vi "Find and Validate Measurement and Device Selection.vi"(8 "error in (no error)":errorcluster, 9 "Device Names":string[](array[string]), 10 "Measurement Name":string, 11 "Controller in":refnum<class "Controller.lvclass">) -> (0 "error out":errorcluster, 1 "Hardware Objects":refnum<class "Hardware.lvclass">[](array[class]), 2 "Measurement out":refnum<class "Measurement.lvclass">, 3 "Controller out":refnum<class "Controller.lvclass">)   [LabVIEW 2015, in "Controller Actor.lvlib" / "Controller.lvclass"]
uses:
  Controller.lvclass
  Hardware/Hardware.lvclass
  Measurement Actor/Measurement.lvclass
panel:
  # "INPUTS"
  # "OUTPUTS"
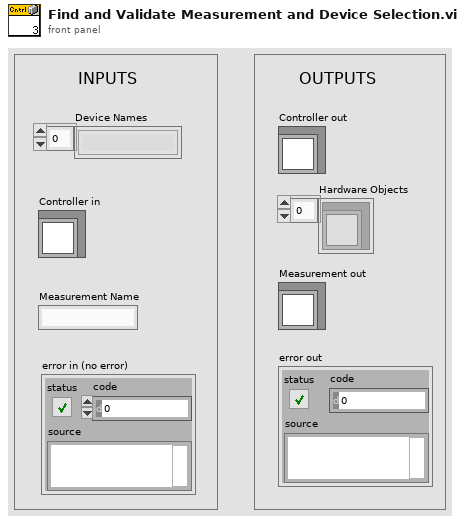
[diagram p1: front panel]
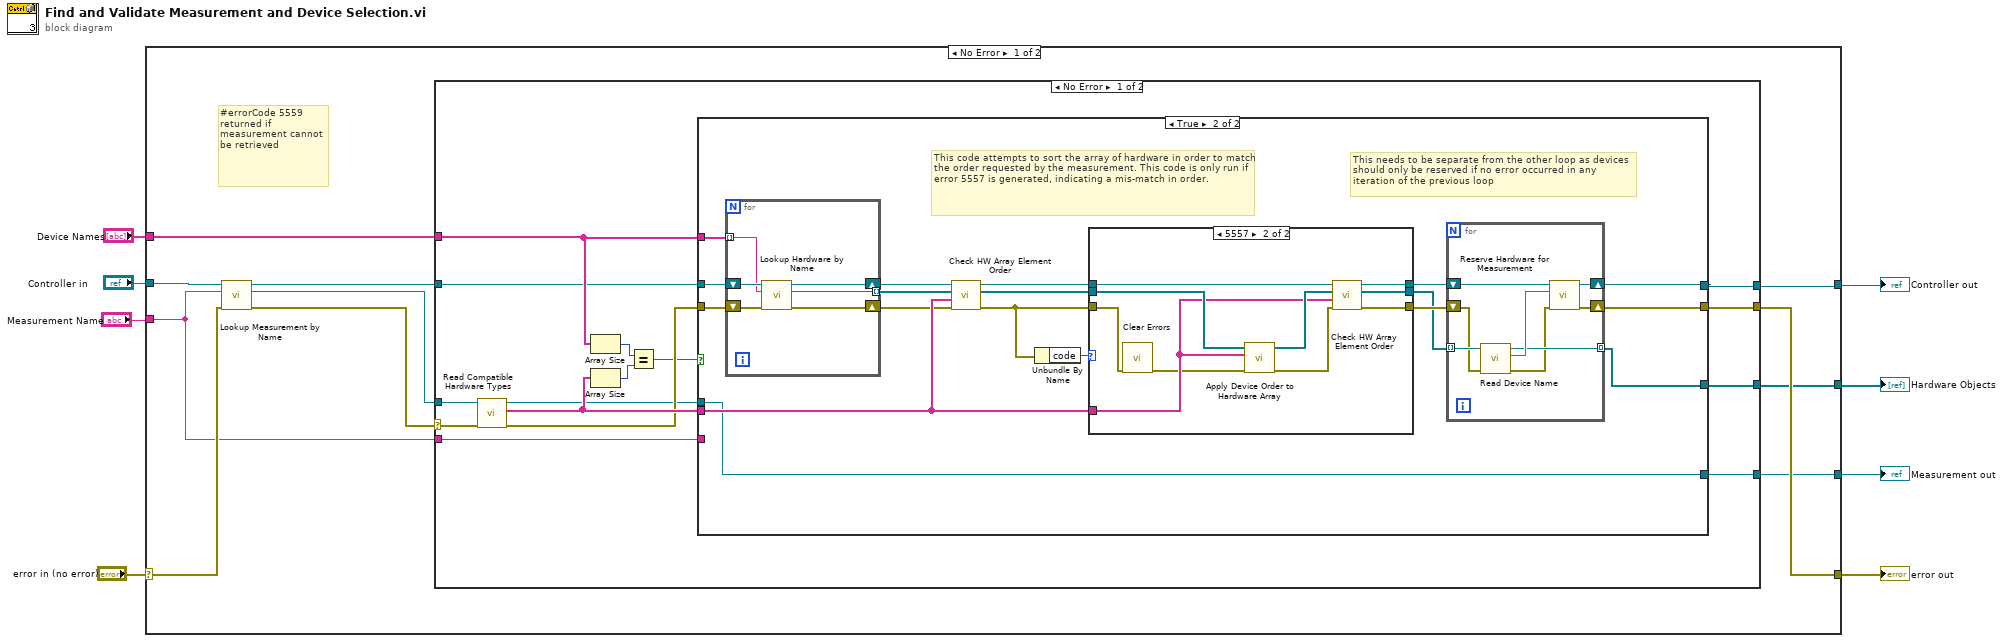
[diagram p0: block diagram]
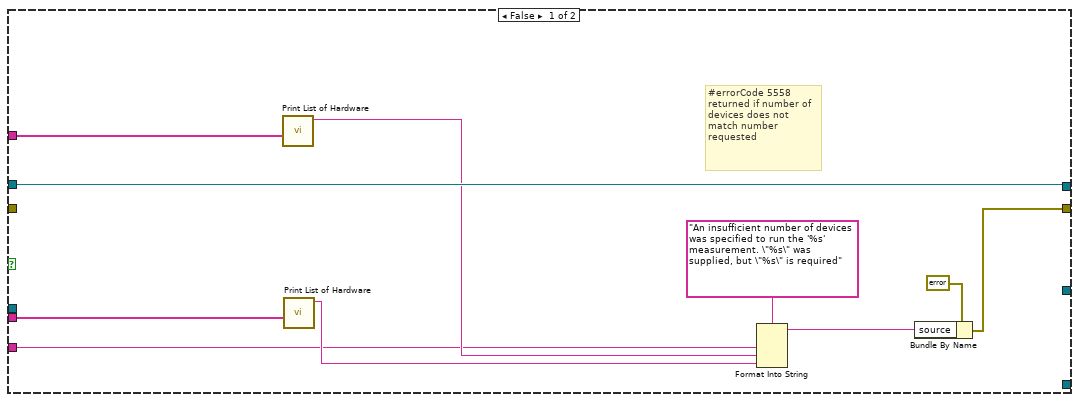
[diagram p2: hidden frame]
diagram:
  n1 = case shown="No Error" "error in (no error)" {
    selector: "error in (no error)" -> [w13 w92]
    tunnel: [w19 w92] -> w8
    tunnel: [w18 w93] -> w7
    tunnel: [w17 _] -> w6
    tunnel: "Controller in" -> [w15 w93]
    tunnel: "Device Names" -> [w16 _]
    tunnel: "Measurement Name" -> [w10 _]
    tunnel: [w11 _] -> w2
    frame No Error {
      # "#errorCode 5559 returned if measurement cannot be retrieved"
      n2 = call "Lookup Measurement by Name.vi"("error in (no error)"=w13, "Measurement Name"=w10, "Controller in"=w15) -> ("error out"=w9:errorcluster, "Measurement.lvclass"=w12:refnum<class "Measurement.lvclass">, "Controller out"=w14:refnum<class "Controller.lvclass">)  [unwired: 5 in, 1 out]
      n3 = case shown="No Error" w9 {
        selector: w9 -> [w20 w91]
        tunnel: [w34 w91] -> w19
        tunnel: [w33 w90] -> w18
        tunnel: [w32 _] -> w17
        tunnel: w16 -> [w31 _]
        tunnel: w14 -> [w25 w90]
        tunnel: w12 -> [w24 _]
        tunnel: [w22 _] -> w11
        tunnel: w10 -> [w21 _]
        frame No Error {
          n4 = call-dynamic "Read Compatible Hardware Types.vi"("error in (no error)"=w20, "Measurement in"=w24) -> ("error out"=w29:errorcluster, "Compatible Hardware Types"=w30:string[], "Measurement out"=w23:refnum<class "Measurement.lvclass">)  [unwired: 7 in]
          n5 = Array Size(array=w31) -> (size(s)=w27:i32)
          n6 = Array Size(array=w30) -> (size(s)=w26:i32)
          n7 = Equal?(x=w27, y=w26) -> (x = y?=w28:bool)
          n8 = case shown="True" w28 {
            tunnel: [w36 w62] -> w34
            tunnel: [w44 w61] -> w33
            tunnel: [_ w49] -> w32
            tunnel: w29 -> [_ w54]
            tunnel: w25 -> [w44 w56]
            tunnel: w31 -> [w43 w57]
            tunnel: w30 -> [w42 w59]
            tunnel: w23 -> [_ w58]
            tunnel: [_ w58] -> w22
            tunnel: w21 -> [w35 _]
            frame False {
              # "#errorCode 5558 returned if number of devices does not match number requested"
              n9 = call "Print List of Hardware.vi"("Device Names"=w43) -> ("String"=w40:string)  [unwired: 10 in]
              n10 = call "Print List of Hardware.vi"("Device Names"=w42) -> ("String"=w39:string)  [unwired: 10 in]
              n11 = Format Into String(format string="An insufficient number of devices was specified to run the '%s' measurement. \"%s\" was supplied, but \"%s\" is required", w35, w40, w39) -> (resulting string=w37:string)  [unwired: 2 in, 1 out]
              n12 = Bundle By Name(cluster=errorcluster {"status"=TRUE, "code"=5558, "source"=""} ("error out"), "source"=w37) -> (w36:errorcluster)
            }
            frame True {
              # "This code attempts to sort the array of hardware in order to match the order requested by the measurement. This code is only run if error 5557 is generated, indicating a mis-match in order."
              # "This needs to be separate from the other loop as devices\nshould only be reserved if no error occurred in any\niteration of the previous loop"
              n13 = for {
                tunnel: w57 -> [w80] mode=indexing
                shift-right: [w79] -> w55
                shift-left: w56 -> [w81]
                shift-right: [w77] -> w53
                shift-left: w54 -> [w78]
                tunnel: [w76] -> w52 mode=indexing
                n14 = call "Lookup Hardware by Name.vi"("error in (no error)"=w78, "Device Name"=w80, "Controller in"=w81) -> ("error out"=w77:errorcluster, "Hardware.lvclass"=w76:refnum<class "Hardware.lvclass">, "Controller out"=w79:refnum<class "Controller.lvclass">)  [unwired: 6 in]
              }
              n15 = call "Check HW Array Element Order.vi"("error in (no error)"=w53, "Compatible Hardware Types"=w59, "Array of Hardware in"=w52, "Controller in"=w55) -> ("error out"=w47:errorcluster, "Array of Hardware out"=w48:refnum<class "Hardware.lvclass">[], "Controller out"=w45:refnum<class "Controller.lvclass">)  [unwired: 5 in]
              n16 = Unbundle By Name(w47) -> ("code"=w46:i32)
              n17 = case shown="5557" w46 {
                tunnel: w59 -> [_ w71]
                tunnel: w48 -> [w64 w75]
                tunnel: [w65 w68] -> w51
                tunnel: w47 -> [w65 w66]
                tunnel: w45 -> [w63 w74]
                tunnel: [w63 w73] -> w60
                tunnel: [w64 w70] -> w50
                frame Default {
                }
                frame 5557 {
                  n18 = call <vilib>:"Clear Errors.vi"("error in (no error)"=w66) -> ("error out"=w67:errorcluster)  [unwired: 5 in, 1 out]
                  n19 = call "Apply Device Order to Hardware Array.vi"("error in (no error)"=w67, "Compatible Hardware Types"=w71, "Array of Hardware in"=w75) -> ("error out"=w69:errorcluster, "Array"=w72:refnum<class "Hardware.lvclass">[])  [unwired: 7 in]
                  n20 = call "Check HW Array Element Order.vi"("error in (no error)"=w69, "Compatible Hardware Types"=w71, "Array of Hardware in"=w72, "Controller in"=w74) -> ("error out"=w68:errorcluster, "Array of Hardware out"=w70:refnum<class "Hardware.lvclass">[], "Controller out"=w73:refnum<class "Controller.lvclass">)  [unwired: 5 in]
                }
              }
              n21 = for {
                shift-right: [w88] -> w61
                shift-left: w60 -> [w89]
                shift-right: [w87] -> w62
                shift-left: w51 -> [w83]
                tunnel: w50 -> [w86] mode=indexing
                tunnel: [w84] -> w49 mode=indexing
                n22 = call "Read Device Name.vi"("error in (no error)"=w83, "Analog in"=w86) -> ("error out"=w82:errorcluster, "Device Name"=w85:string, "Analog out"=w84:refnum<class "Hardware.lvclass">)  [unwired: 7 in]
                n23 = call "Reserve Hardware for Measurement.vi"("error in (no error)"=w82, "Hardware to Reserve"=w85, "Controller in"=w89) -> ("error out"=w87:errorcluster, "Controller out"=w88:refnum<class "Controller.lvclass">)  [unwired: 7 in]
              }
            }
          }
        }
        frame Error {
        }
      }
    }
    frame Error {
    }
  }
  "error out" <- w8
  "Controller out" <- w7
  "Hardware Objects" <- w6
  "Measurement out" <- w2
